vi "WeatherStationMain_20180517.vi"() -> ()   [LabVIEW 2018]
doc: "Logs and displays weather data in real-time from the Vaisala WXT520 Weather Station and the Optical Scientific ORG-815 Optical Rain Gauge."
uses:
  Weather_UserConfig_Clust.ctl
  Epimedia_Connex_Source/Controls/Enums/WatchdogTimer_Enum.ctl
  Epimedia_Connex_Source/Controls/Clusts/WeatherDataClust.ctl
  Epimedia_Connex_Source/Controls/Clusts/ValidityWeatherClust.ctl
  Epimedia_Connex_Source/Controls/Enums/LogLoopEnum.ctl
  <vilib>/Analysis/baseanly.llb/Mean (DBL).vi
  <vilib>/Analysis/NI_AALBase.lvlib
  <vilib>/ptbypt/NI_PtbyPt.lvlib
panel:
  out "Wind Gusts":dbl format="%.3g"
  in  "Port":refnum<visa-resource-name>="Port3"
  out "Wind Direction":dbl format="%.3g"
  out "Wind Speed":dbl format="%.3g"
  out "Pressure":dbl format="%.3g"
  out "Humidity":dbl format="%.3g"
  out "Temperature":dbl format="%.3g"
  out "Running LED":bool
  out "Uptime":string="00:00:00"
  out "Progress Bar":u32(slide) scale=0.0..60.0
  in  "stop":bool
  out "Rain Fall":dbl format="%.3g"
  out "Rain Rate":dbl format="%.3g"
  out "Warning":string
  out "Plot 3":cluster{"array":dbl[], "array":dbl[]}[](graph)
  out "Plot 2":cluster{"array":dbl[], "array":dbl[]}[](graph)
  out "Plot 1":cluster{"array":dbl[], "array":dbl[]}[](graph)
  out "Young Error":bool
  out "Young":T1
  # "Port"
  # "CONDITIONS"
  # "mm / hr"
  # "mm"
  # "°C"
  # "%"
  # "mBar"
  # "m / s"
  # "°"
  # "m / s"
  # "Recording"
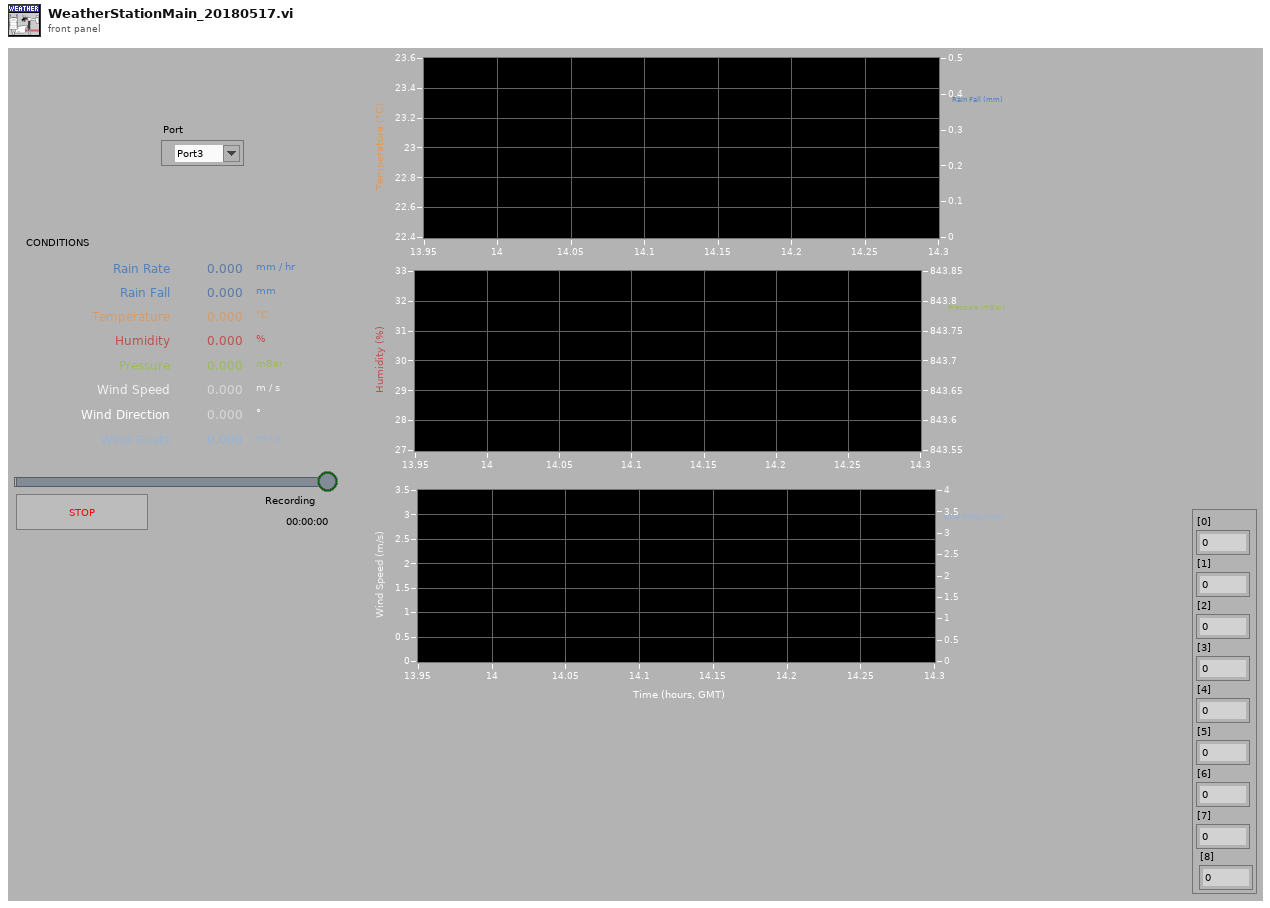
[diagram p1: front panel]
types:
  T1 = cluster{"[0]":dbl, "[1]":dbl, "[2]":dbl, "[3]":dbl, "[4]":dbl, "[5]":dbl, "[6]":dbl, "[7]":dbl, "[8]":dbl}
  T2 = typedef "Weather_UserConfig_Clust.ctl" = cluster{"Port":refnum<visa-resource-name>}
  T3 = cluster{"[0]":dbl, "[1]":dbl, "[2]":dbl, "[3]":dbl, "[4]":dbl, "[5]":dbl, "[6]":dbl, "[7]":dbl}
  T4 = cluster{"[0]":dbl, dbl, "[1]":dbl, "[2]":dbl, "[3]":dbl, "[4]":dbl, dbl, "[6]":dbl, dbl}
  T5 = typedef "WatchdogTimer_Enum.ctl" = enum16{"ResetAll", "CheckAll", "HW1", "HW2", "Tones", "FP", "Noise", "Log", "TCP", "AI", "TC", "ADAM", "Disdrom", "TE", "Weather"}
  T6 = typedef "LogLoopEnum.ctl" = enum16{"Log_Init", "Log_Config", "Log_CfgAlarm", "Log_TimeDomain", "Log_Tone", "Log_NoiseTrace", "Log_NoiseSum", "Log_DO", "Log_AI", "Log_TC", "Log_Disdrom", "Log_Weather", "Log_TE", "Log_ADAM", "Log_UPS", "Log_ChkTime", "Log_Alarm", "Log_SSH", "Log_Write", "Log_Exit"}
  T7 = typedef "WeatherDataClust.ctl" = cluster{"TimeString":string, "Timestamp":dbl, "Wind Speed":sgl, "Wind Gusts":sgl, "Wind Dir":sgl, "Wind Dir STD":sgl, "Temperature":sgl, "Humidity":sgl, "Pressure":sgl, "Rain Rate":i16, "Rain Fall":sgl, "Status":T8}
  T8 = typedef "ValidityWeatherClust.ctl" = cluster{"Temp_OutOfBounds":bool, "Temp_IncrSTD":bool, "Temp_Oth":bool, "BarPress_OutOfBounds":bool, "BarPress_IncrSTD":bool, "BarPress_Change":bool, "BarPress_Other":bool, "Humid_OutOfBounds":bool, "Humid_IncrSTD":bool, "Humid_Other":bool, "Wind__Spd_OutOfBounds":bool, "Wind_Dir_OutOfBounds":bool, "RainBuck_OutOfBounds":bool, "RainBuck_Disdrom":bool, "Disdrom_RainBuck":bool, "Placeholder":bool}
  T9 = cluster{"Timestamp":dbl[], "ORG Rain Fall":dbl[]}[]
  T10 = cluster{"Timestamp":dbl[], "WXT Pressure":dbl[]}[]
  T11 = cluster{"Timestamp":dbl[], "WXT Wind Direction":dbl[]}[]
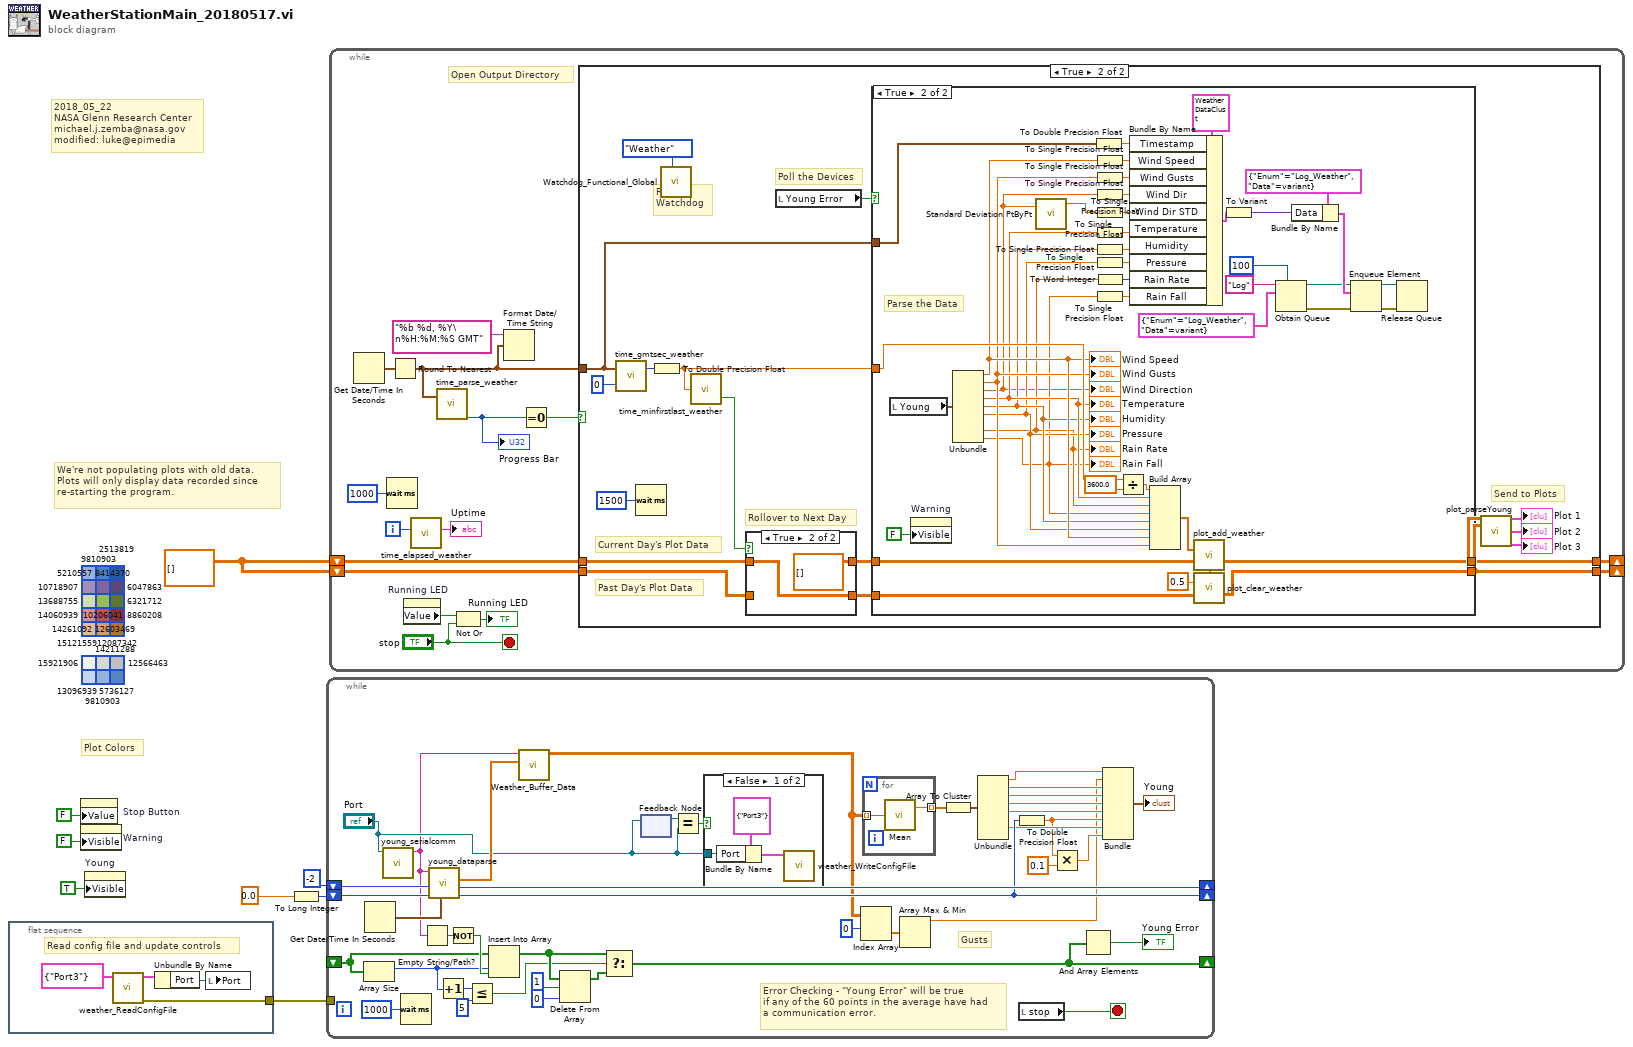
[diagram p0: block diagram]
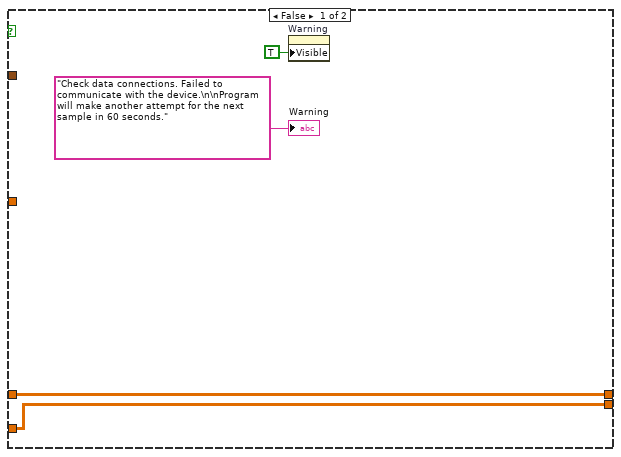
[diagram p4: hidden frame]
diagram:
  w5 = dbl[][] [] ("Loaded Data Array")
  (unwired) u32 6321712
  (unwired) u32 8860208
  (unwired) u32 12087342
  (unwired) u32 12566463
  (unwired) u32 5736127
  (unwired) u32 14060939
  (unwired) u32 15121559
  (unwired) u32 15921906
  (unwired) u32 13096939
  (unwired) u32 13688755
  (unwired) u32 6047863
  (unwired) u32 10718907
  (unwired) u32 9810903
  (unwired) u32 10206041
  (unwired) u32 8414370
  (unwired) u32 12603469
  (unwired) u32 14261092
  (unwired) u32 14211288
  (unwired) u32 9810903
  (unwired) u32 2513819
  (unwired) u32 5210557
  # "We're not populating plots with old data.\nPlots will only display data recorded since \nre-starting the program."
  # "2018_05_22\nNASA Glenn Research Center\nmichael.j.zemba@nasa.gov\nmodified: luke@epimedia"
  # "Plot Colors"
  n1 = flat-sequence {
    tunnel: [w11] -> w1
    frame #0 {
      # "Read config file and update controls"
      n2 = call "weather_ReadConfigFile.vi"("User"=T2 {"Port"="Port3"}) -> ("ErrorOut"=w11:errorcluster, "User"=w10:T2)  [unwired: 8 in, 1 out]
      n3 = Unbundle By Name(w10) -> ("Port"=w9:refnum<visa-resource-name>)
      n4 = local write "Port"(w9) -> ()
    }
  }
  n5 = property on="Stop Button" class="Bool (strict)"("Value"=FALSE ("Visible")) -> ()  [unwired: 2 in, 2 out]
  n6 = property on="Warning" class="Str"("Visible"=FALSE) -> ()  [unwired: 2 in, 2 out]
  n7 = property on="Young" class="Clust (strict)"("Visible"=TRUE) -> ()  [unwired: 2 in, 2 out]
  n8 = To Long Integer(number=0.0 ("Last Tips Value")) -> (32bit integer=w4:i32)
  n9 = while {
    shift-right: [w51] -> _
    shift-left: -2 ("TB Out") -> [w53]
    shift-right: [w43] -> _
    shift-left: w4 -> [w52]
    shift-right: [w33] -> _
    shift-left: _ -> [w40]
    tunnel: w1 -> [_]
    stop <- w48 stop-if-true
    # "Gusts"
    # "Error Checking - \"Young Error\" will be true\nif any of the 60 points in the average have had\na communication error."
    n10 = Array Size(array=w40) -> (size(s)=w38:i32)
    n11 = Get Date/Time In Seconds() -> (seconds since 1Jan1904=w29:timestamp)
    n12 = call "young_serialcomm.vi"("Resource Name"="Port") -> ("Poll Response"=w14:string)  [unwired: 8 in, 2 out]
    n13 = Wait (ms)(milliseconds to wait=u32 1000) -> ()  [unwired: 1 out]
    n14 = Empty String/Path?(string/path=w14) -> (empty?=w42:bool)
    n15 = call "young_dataparse.vi"("Current Time"=w29, "Tips In"=w52, "TB In"=w53, "Poll Response"=w14) -> ("Tips Out"=w43:i32, "TB Out"=w51:i32, "Output Array"=w50:dbl[])  [unwired: 5 in]
    n16 = Increment(x=w38) -> (x+1=w39:i32)
    n17 = Not(x=w42) -> (.not. x?=w41:bool)
    n18 = Less Or Equal?(x=w39, y=5) -> (x <= y?=w34:bool)
    n19 = Insert Into Array(array=w40, index=w38, new element=w41) -> (w36:bool[])
    n20 = call "Weather_Buffer_Data.vi"("Parsed Data Array"=w50, "Un-Parsed String"=w14) -> ("Plot Arrays"=w13:dbl[][])  [unwired: 9 in]
    n21 = Delete From Array(array=w36, length=1, index=0) -> (array with subset deleted=w35:bool[])  [unwired: 1 out]
    n22 = Select(t=w36, s=w34, f=w35) -> (s? t:f=w33:bool[])
    n23 = feedback-in #1("Port") -> ()
    n24 = feedback #1() -> (w17:refnum<visa-resource-name>)  [unwired: 1 in]
    n25 = Equal?(x=w17, y="Port") -> (x = y?=w15:bool)
    n26 = case shown="False" w15 {
      tunnel: "Port" -> [w54 _]
      frame False {
        n27 = Bundle By Name(cluster=T2 {"Port"="Port3"} ("User"), "Port"=w54) -> (w55:T2)
        n28 = call "weather_WriteConfigFile.vi"("User"=w55) -> ()  [unwired: 10 in, 1 out]
      }
      frame True {
      }
    }
    n29 = Index Array(array=w13, index (row)=0) -> (element=w27:dbl[])  [unwired: 1 in]
    n30 = for {
      tunnel: w13 -> [w58] mode=indexing
      tunnel: [w57] -> w49 mode=indexing
      n31 = call-poly <vilib>:"Mean.vi"("X"=w58) -> ("mean"=w57:dbl)  [unwired: 1 out]
    }
    n32 = Array Max & Min(array=w27) -> (max value=w19:dbl)  [unwired: 3 out]
    n33 = Array To Cluster(array=w49) -> (cluster=w46:T3)
    n34 = Unbundle(w46) -> ("[0]"=w45:dbl, "[1]"=w20:dbl, "[2]"=w21:dbl, "[3]"=w22:dbl, "[4]"=w23:dbl, "[6]"=w25:dbl)  [unwired: 2 out]
    n35 = To Double Precision Float(number=w43) -> (double precision float=w24:dbl)
    n36 = local read "stop"() -> (w48:bool)
    n37 = Multiply(x=w24, y=0.1) -> (x*y=w26:dbl)
    n38 = And Array Elements(Boolean array=w33) -> (logical AND=→"Young Error":bool)
    n39 = Bundle("[0]"=w45, w19, "[1]"=w20, "[2]"=w21, "[3]"=w22, "[4]"=w23, w24, "[6]"=w25, w26) -> (→"Young":T4)  [unwired: 1 in]
  }
  n40 = while {
    shift-right: [w67] -> _
    shift-left: w5 -> [w66]
    shift-right: [w64] -> _
    shift-left: w5 -> [w65]
    i -> [w59]
    stop <- "stop" stop-if-true
    # "Open Output Directory"
    n41 = Get Date/Time In Seconds() -> (seconds since 1Jan1904=w61:timestamp)
    n42 = Wait (ms)(milliseconds to wait=u32 1000) -> ()  [unwired: 1 out]
    n43 = Round To Nearest(number=w61) -> (nearest integer value=w60:timestamp)
    n44 = property on="Running LED" class="Bool (strict)"() -> ("Value"=w73:bool)  [unwired: 2 in, 2 out]
    n45 = call "time_elapsed_weather.vi"("Elapsed Time (sec)"=w59) -> ("Elapsed Time (string)"=→"Uptime":string)  [unwired: 10 in]
    n46 = call "time_parse_weather.vi"("Current Time"=w60) -> ("Seconds"=w62:u32)  [unwired: 12 in, 6 out]
    "Progress Bar" <- w62
    n47 = Not Or(1:"stop", 2:w73) -> (0:→"Running LED":bool)
    n48 = Format Date/Time String(time format string (%c)="%b %d, %Y\n%H:%M:%S GMT", seconds (now)=w60) -> ()  [unwired: 1 in, 1 out]
    n49 = Equal To 0?(x=w62) -> (x = 0?=w71:bool)
    n50 = case shown="True" w71 {
      tunnel: w60 -> [_ w76]
      tunnel: [w75 w83] -> w67
      tunnel: w66 -> [w75 w92]
      tunnel: w65 -> [w74 w91]
      tunnel: [w74 w84] -> w64
      frame False {
      }
      frame True {
        # "Reset\nWatchdog"
        # "Send to Plots"
        # "Current Day's Plot Data"
        # "Past Day's Plot Data"
        # "Poll the Devices"
        # "Rollover to Next Day"
        n51 = call "time_gmtsec_weather.vi"("Timezone Offset (Hrs)"=0, "Timestamp"=w76) -> ("Sec Since 12AM GMT"=w80:u32)  [unwired: 1 out]
        n52 = Wait (ms)(milliseconds to wait=u32 1500) -> ()  [unwired: 1 out]
        n53 = To Double Precision Float(number=w80) -> (double precision float=w79:dbl)
        n54 = call "Watchdog_Functional_Global.vi"("Watchdog"=WatchdogTimer_Enum."Weather") -> ()  [unwired: 9 in, 2 out]
        n55 = call "time_minfirstlast_weather.vi"("Sec. from Midnight"=w79) -> ("First Minute of Day"=w88:bool)  [unwired: 2 in, 1 out]
        n56 = case shown="True" w88 {
          tunnel: w92 -> [w142 w144]
          tunnel: [w142 dbl[][] [] ("Input Arrays")] -> w90
          tunnel: [w141 w144] -> w89
          tunnel: w91 -> [w141 _]
          frame False {
          }
          frame True {
          }
        }
        n57 = local read "Young Error"() -> (w82:bool)
        n58 = case shown="True" w82 {
          tunnel: w79 -> [_ w128]
          tunnel: w90 -> [w96 w136]
          tunnel: [w96 w135] -> w83
          tunnel: w89 -> [w95 w137]
          tunnel: [w95 w134] -> w84
          tunnel: w76 -> [_ w97]
          frame False {
            n59 = property on="Warning" class="Str"("Visible"=TRUE) -> ()  [unwired: 2 in, 2 out]
            "Warning" <- "Check data connections. Failed to communicate with the device.\n\nProgram will make another attempt for the next sample in 60 seconds."
          }
          frame True {
            # "Parse the Data"
            n60 = local read "Young"() -> (w130:T1)
            n61 = property on="Warning" class="Str"("Visible"=FALSE) -> ()  [unwired: 2 in, 2 out]
            n62 = Unbundle(w130) -> ("[0]"=w127:dbl, "[1]"=w115:dbl, "[2]"=w101:dbl, "[3]"=w114:dbl, "[4]"=w113:dbl, "[5]"=w112:dbl, "[7]"=w111:dbl, "[8]"=w110:dbl)  [unwired: 1 out]
            "Rain Rate" <- w111
            "Rain Fall" <- w110
            "Temperature" <- w114
            "Humidity" <- w113
            "Pressure" <- w112
            "Wind Speed" <- w127
            "Wind Direction" <- w101
            "Wind Gusts" <- w115
            n63 = call <vilib>:"Standard Deviation PtByPt.vi"("x"=w101) -> ("standard deviation"=w99:dbl)  [unwired: 2 in, 2 out]
            n64 = To Double Precision Float(number=w97) -> (double precision float=w98:dbl)
            n65 = To Single Precision Float(number=w127) -> (single precision float=w109:sgl)
            n66 = To Single Precision Float(number=w115) -> (single precision float=w108:sgl)
            n67 = To Single Precision Float(number=w101) -> (single precision float=w107:sgl)
            n68 = To Single Precision Float(number=w99) -> (single precision float=w100:sgl)
            n69 = To Single Precision Float(number=w114) -> (single precision float=w106:sgl)
            n70 = To Single Precision Float(number=w113) -> (single precision float=w105:sgl)
            n71 = To Single Precision Float(number=w112) -> (single precision float=w104:sgl)
            n72 = To Word Integer(number=w111) -> (16bit integer=w103:i16)
            n73 = To Single Precision Float(number=w110) -> (single precision float=w102:sgl)
            n74 = Divide(x=w128, y=3600.0) -> (x/y=w133:dbl)
            n75 = Bundle By Name(cluster=T7 {"TimeString"="", "Timestamp"=0.0, "Wind Speed"=0.0, "Wind Gusts"=0.0, "Wind Dir"=0.0, "Wind Dir STD"=0.0, "Temperature"=0.0, "Humidity"=0.0, "Pressure"=0.0, "Rain Rate"=0, "Rain Fall"=0.0, "Status"={"Temp_OutOfBounds"=FALSE, "Temp_IncrSTD"=FALSE, "Temp_Oth"=FALSE, "BarPress_OutOfBounds"=FALSE, "BarPress_IncrSTD"=FALSE, "BarPress_Change"=FALSE, "BarPress_Other"=FALSE, "Humid_OutOfBounds"=FALSE, "Humid_IncrSTD"=FALSE, "Humid_Other"=FALSE, "Wind__Spd_OutOfBounds"=FALSE, "Wind_Dir_OutOfBounds"=FALSE, "RainBuck_OutOfBounds"=FALSE, "RainBuck_Disdrom"=FALSE, "Disdrom_RainBuck"=FALSE, "Placeholder"=FALSE}}, "Timestamp"=w98, "Wind Speed"=w109, "Wind Gusts"=w108, "Wind Dir"=w107, "Wind Dir STD"=w100, "Temperature"=w106, "Humidity"=w105, "Pressure"=w104, "Rain Rate"=w103, "Rain Fall"=w102) -> (w116:T7)
            n76 = Build Array(w133, w114, w111, w110, w113, w112, w127, w115) -> (w138:dbl[])
            n77 = call "plot_add_weather.vi"("Input Points"=w138, "Input Arrays"=w136) -> ("Output Arrays"=w135:dbl[][], "Timestamps"=w140:dbl[])  [unwired: 12 in]
            n78 = call "plot_clear_weather.vi"("Clearing Array"=w140, "Buffer Size"=0.5, "Input Arrays"=w137) -> ("Output Arrays"=w134:dbl[][])  [unwired: 12 in]
            n79 = To Variant(anything=w116) -> (Variant=w117:variant)
            n80 = Obtain Queue(max queue size (-1, unlimited)=100, name (unnamed)="Log", element data type=cluster{"Enum":T6, "Data":variant} {"Enum"=enum."Log_Weather", "Data"=variant}) -> (queue out=w121:refnum<queue>, error out=w122:errorcluster)  [unwired: 2 in, 1 out]
            n81 = Bundle By Name(cluster=cluster{"Enum":T6, "Data":variant} {"Enum"=enum."Log_Weather", "Data"=variant}, "Data"=w117) -> (w123:cluster{"Enum":T6, "Data":variant})
            n82 = Enqueue Element(queue=w121, element=w123, error in (no error)=w122) -> (queue out=w124:refnum<queue>, error out=w125:errorcluster)  [unwired: 1 in, 1 out]
            n83 = Release Queue(queue=w124, error in (no error)=w125) -> ()  [unwired: 1 in, 3 out]
          }
        }
        n84 = call "plot_parseYoung.vi"("Current Data"=w83, "Yesterday's Data"=w84) -> ("Plot 1"=→"Plot 1":T9, "Plot 2"=→"Plot 2":T10, "Plot 3"=→"Plot 3":T11)  [unwired: 11 in]
      }
    }
  }
